vi "T13 - Калибровка входа АЦП.vi"() -> ()   [LabVIEW 2009]
uses:
  Z210/Z210 CTL Lib.llb/Z210 CTL ADC Linear Correction.ctl
  Z210/Z210 CTL Lib.llb/Z210 CTL ADC or DAC Function.ctl
  Instance          12 34Saved   T13 - Калибровка входа АЦП .vi
  <vilib>/Analysis/NI_AALPro.lvlib
panel:
  in  "Linear Correction ADC":T1=[{"scale"=1.0, "offset"=0.0}, {"scale"=1.0, "offset"=0.0}, {"scale"=1.0, "offset"=0.0}, {"scale"=1.0, "offset"=0.0}, {"scale"=1.0, "offset"=0.0}, {"scale"=1.0, "offset"=0.0}, {"scale"=1.0, "offset"=0.0}, {"scale"=1.0, "offset"=0.0}, {"scale"=1.0, "offset"=0.0}, {"scale"=1.0, "offset"=0.0}, {"scale"=1.0, "offset"=0.0}, {"scale"=1.0, "offset"=0.0}, {"scale"=1.0, "offset"=0.0}, {"scale"=1.0, "offset"=0.0}, {"scale"=1.0, "offset"=0.0}, {"scale"=1.0, "offset"=0.0}]
  out "C коррекцией":dbl[unit][](array[numeric])
  out "без коррекции":dbl[unit][](array[numeric])
  in  "Points":i32=6
  out "XY Graph":cluster{dbl[], dbl[]}[](graph)
  out "mse":dbl format="%.12g"
  out "intercept":dbl format="%.12g"
  out "slope":dbl format="%.12g"
  out "Поверенные":dbl[](array[numeric])
  # "Калибровка и коррекция напряжения по входу АЦП#0"
  # "Позволяет откалибровать значения напряжений, записываемых с входа АЦП #0  по поверенному вольтметру.\nИзмеряется напряжение в нескольких точках, линейно аппроксимируется, высчитываются поправочные коэффициенты."
  # "1. Соединить АЦП#0 и ЦАП#0. Туда же повесить вольтметр.\n2. Установить число точек контрольных измерений (не менее 2).\n3. Запустить. Ввести поверенные значения.\n4. Посмотреть на коэфф. коррекции и сравнить 1й и 3й столбик напряжений"
  # "Напряжения"
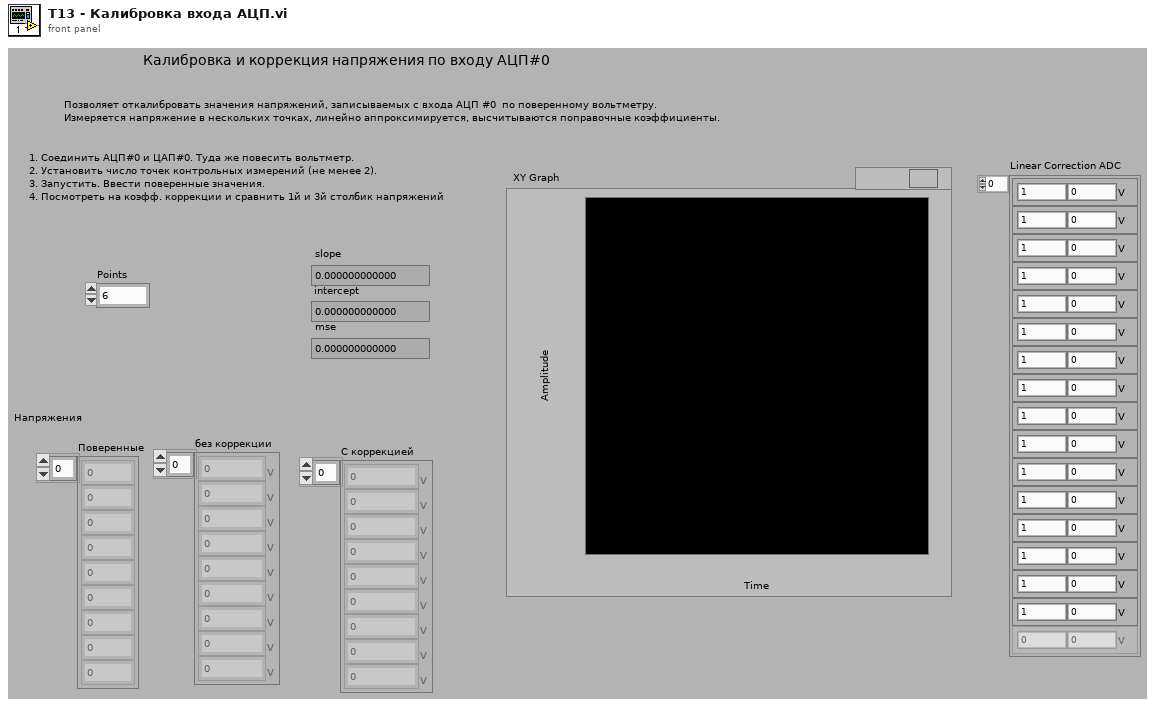
[diagram p1: front panel]
types:
  T1 = typedef "Z210 CTL ADC Linear Correction.ctl" = cluster{"scale":dbl, "offset":dbl[unit]}[]
  T2 = typedef "Z210 CTL ADC or DAC Function.ctl" = enum16{"АЦП", "ЦАП", "Both"}
  T3 = typedef "Z210 CTL Unit Data .ctl" = cluster{"typeDevice":i32, "numberDSP":i32}
  T4 = typedef "Z210 CTL Buffers Params.ctl" = cluster{"bufferAddr ADC":u32, "bufferSize ADC":i32, "bufferAddr DAC":u32, "bufferSize DAC":i32}
  T5 = typedef "Z210 CTL ADC Voltages.ctl" = dbl[unit][]
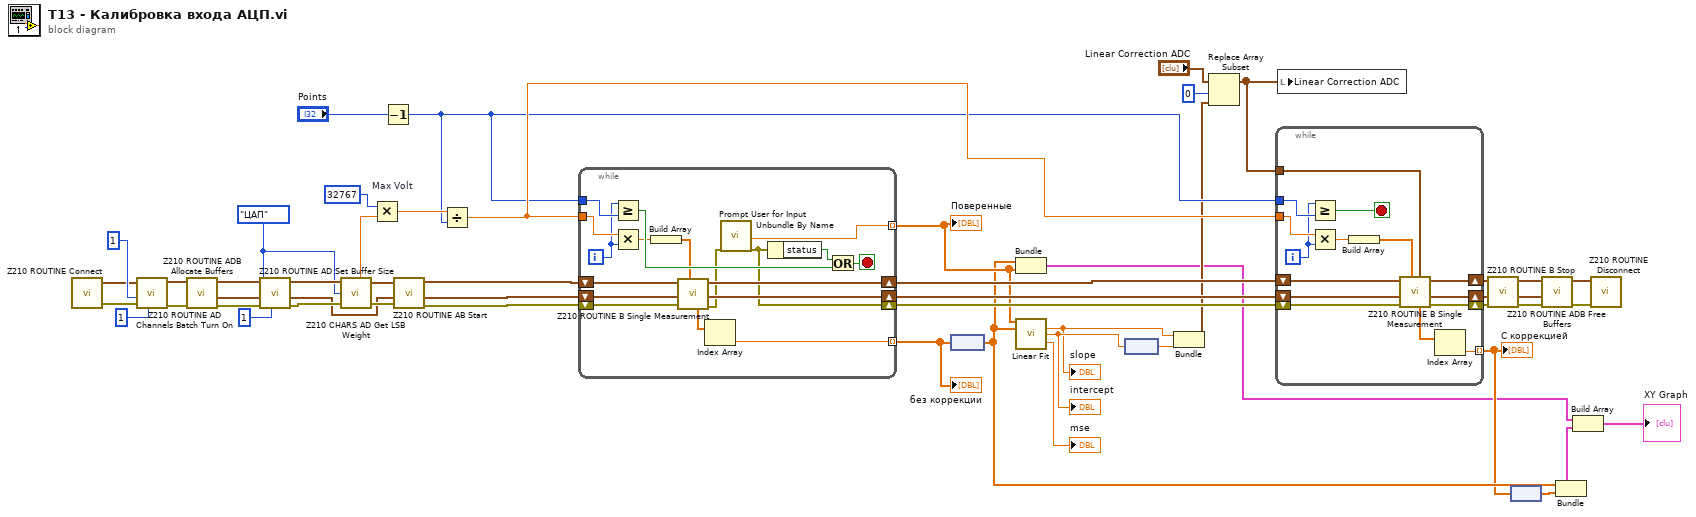
[diagram p0: block diagram]
diagram:
  w29 = Z210_CTL_ADC_or_DAC_Function."ЦАП" ("AorD")
  n1 = call "Z210 ROUTINE Connect.vi"() -> ("error out"=w27:errorcluster, "unitData out"=w28:T3)  [unwired: 10 in]
  n2 = call "Z210 ROUTINE AD Channels Batch Turn On.vi"("N ЦАП (0)"=1, "error in (no error)"=w27, "N Синф (0)"=1, "unitData in"=w28) -> ("error out"=w36:errorcluster, "unitData out"=w37:T3)  [unwired: 4 in, 2 out]
  n3 = call "Z210 ROUTINE ADB Allocate Buffers.vi"("error in (no error)"=w36, "unitData in"=w37) -> ("error out"=w47:errorcluster, "buffersParams out"=w49:T4, "unitData out"=w48:T3)  [unwired: 7 in]
  n4 = call "Z210 ROUTINE AD Set Buffer Size.vi"("size suggestion (0)"=1, "error in (no error)"=w47, "buffersParams"=w49, "AorD"=w29, "unitData in"=w48) -> ("error out"=w45:errorcluster, "buffersParams out"=w38:T4, "unitData out"=w46:T3)  [unwired: 3 in, 1 out]
  n5 = call "Z210 CHARS AD Get LSB Weight.vi"("unitData in"=w46, "AorD"=w29, "error in (no error)"=w45) -> ("LBSweight"=w43:dbl[unit], "unitData out"=w40:T3, "error out"=w39:errorcluster)  [unwired: 4 in]
  n6 = Multiply "Max Volt"(x=i16 32767, y=w43) -> (x*y=w42:dbl[unit])
  n7 = Decrement(x="Points") -> (x-1=w33:i32)
  n8 = call "Z210 ROUTINE AB Start.vi"("error in (no error)"=w39, "buffersParams"=w38, "unitData in"=w40) -> ("error out"=w1:errorcluster, "buffersParams out"=w50:T4, "unitData out"=w51:T3)  [unwired: 6 in]
  n9 = Divide(x=w42, y=w33) -> (x/y=w41:dbl[unit])
  n10 = while {
    tunnel: w33 -> [w69]
    shift-right: [w55] -> w15
    shift-left: w1 -> [w62]
    shift-right: [w59] -> w16
    shift-left: w50 -> [w61]
    shift-right: [w58] -> w17
    shift-left: w51 -> [w63]
    tunnel: w41 -> [w70]
    tunnel: [w64] -> w19 mode=indexing
    tunnel: [w56] -> w14 mode=indexing
    i -> [w65]
    stop <- w68 stop-if-true
    n11 = Greater Or Equal?(x=w65, y=w69) -> (x >= y?=w66:bool)
    n12 = Multiply(x=w70, y=w65) -> (x*y=w53:dbl[unit])
    n13 = Build Array(w53) -> (w54:dbl[unit][])
    n14 = call "Z210 ROUTINE B Single Measurement.vi"("DAC Voltages"=w54, "error in (no error)"=w62, "buffersParams"=w61, "unitData in"=w63) -> ("error out"=w57:errorcluster, "buffersParams out"=w59:T4, "unitData out"=w58:T3, "ADC Voltages"=w60:T5)  [unwired: 4 in]
    n15 = Index Array(array=w60) -> (element=w64:dbl[unit])  [unwired: 1 in]
    n16 = call "Prompt User for Input"("error in (no error)"=w57) -> ("calibratedVoltage"=w56:dbl, "error out"=w55:errorcluster)  [unwired: 16 in, 1 out]
    n17 = Unbundle By Name(w55) -> ("status"=w67:bool)
    n18 = Or(x=w67, y=w66) -> (x .or. y?=w68:bool)
  }
  "Поверенные" <- w14
  "без коррекции" <- w19
  n19 = node(w19) -> (w7:dbl[])
  n20 = Bundle(w7, w14) -> (w4:cluster{dbl[], dbl[]})  [unwired: 1 in]
  n21 = call <vilib>:"Linear Fit.vi"("Y"=w14, "X"=w7) -> ("slope"=w10:dbl, "intercept"=w18:dbl, "residue"=→"mse":dbl)  [unwired: 9 in, 2 out]
  "slope" <- w10
  "intercept" <- w18
  n22 = node(w18) -> (w11:dbl[unit])
  n23 = Bundle("slope"=w10, w11) -> (w9:cluster{"slope":dbl, dbl[unit]})  [unwired: 1 in]
  n24 = Replace Array Subset(array="Linear Correction ADC", new element=w9, index=0) -> (w8:T1)
  n25 = while {
    tunnel: w33 -> [w84]
    shift-right: [w74] -> w32
    shift-left: w15 -> [w79]
    shift-right: [w71] -> w31
    shift-left: w16 -> [w80]
    shift-right: [w81] -> w30
    shift-left: w17 -> [w82]
    tunnel: w41 -> [w85]
    tunnel: w8 -> [w76]
    tunnel: [w72] -> w6 mode=indexing
    i -> [w83]
    stop <- w75 stop-if-true
    n26 = Greater Or Equal?(x=w83, y=w84) -> (x >= y?=w75:bool)
    n27 = Multiply(x=w85, y=w83) -> (x*y=w78:dbl[unit])
    n28 = Build Array(w78) -> (w77:dbl[unit][])
    n29 = call "Z210 ROUTINE B Single Measurement.vi"("Linear Correction ADC"=w76, "DAC Voltages"=w77, "error in (no error)"=w79, "buffersParams"=w80, "unitData in"=w82) -> ("error out"=w74:errorcluster, "buffersParams out"=w71:T4, "unitData out"=w81:T3, "ADC Voltages"=w73:T5)  [unwired: 3 in]
    n30 = Index Array(array=w73) -> (element=w72:dbl[unit])  [unwired: 1 in]
  }
  "C коррекцией" <- w6
  n31 = local write "Linear Correction ADC"(w8) -> ()
  n32 = call "Z210 ROUTINE B Stop.vi"("error in (no error)"=w32, "buffersParams"=w31, "unitData in"=w30) -> ("error out"=w23:errorcluster, "buffersParams out"=w22:T4, "unitData out"=w25:T3)  [unwired: 6 in]
  n33 = node(w6) -> (w3:dbl[])
  n34 = call "Z210 ROUTINE ADB Free Buffers.vi"("error in (no error)"=w23, "buffersParams"=w22, "unitData in"=w25) -> ("error out"=w21:errorcluster, "unitData out"=w24:T3)  [unwired: 6 in, 1 out]
  n35 = Bundle(w7, w3) -> (w5:cluster{dbl[], dbl[]})  [unwired: 1 in]
  n36 = Build Array(w4, w5) -> (→"XY Graph":cluster{dbl[], dbl[]}[])
  n37 = call "Z210 ROUTINE Disconnect.vi"("error in (no error)"=w21, "unitData in"=w24) -> ()  [unwired: 8 in, 2 out]
